vi "Create.vi"(8 "error in (no error)":errorcluster, 10 "EnQr":refnum<class "Message Enqueuer.lvclass">) -> (0 "error out":errorcluster, 3 "LoggingAPI out":refnum<class "LoggingAPI.lvclass">)   [LabVIEW 2020, in "Volatus.lvlib" / "LoggingAPI.lvclass"]
uses:
  LoggingAPI.lvclass
  <vilib>/ActorFramework/Message Enqueuer/Message Enqueuer.lvclass
  LoggingAPI.lvclass/LoggingAPI.ctl
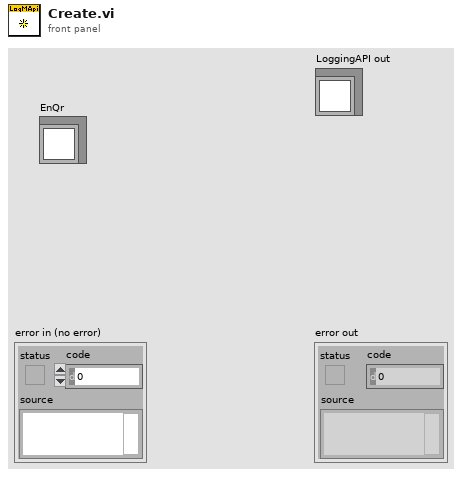
[diagram p1: front panel]
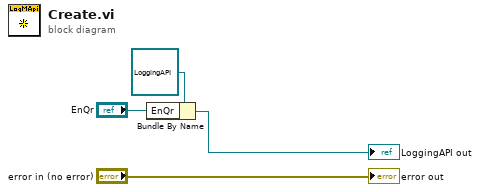
[diagram p0: block diagram]
diagram:
  n1 = Bundle By Name(cluster=refnum<class "LoggingAPI.lvclass"> refnum ("LoggingAPI in"), "EnQr"="EnQr") -> (→"LoggingAPI out":refnum<class "LoggingAPI.lvclass">)
  "error out" <- "error in (no error)"
